vi "Advanced Serial Write and Read.vi"(0 "VISA resource name":refnum<visa-resource-name>="COM1", 1 "baud rate":u32=9600, 3 "bytes to read":u32=1000, 4 "data bits":u16=8 min=5 max=8 step=1, 5 "parity":u16(ring) items=["None", "Odd", "Even", "Mark", "Space"], 7 "stop bits":u16(ring)=10 items=["1.0"=10, "1.5"=15, "2.0"=20], 9 "XON Character":u8=17 format="%.0x", 13 "string to write":string="*IDN?", 14 "XOFF Character":u8=19 format="%.0x", 15 "timeout (ms)":u32=10000, 17 "write":bool=TRUE, 21 "End read on termination character?":bool=TRUE, 24 "termination char\n(0xA = '\\n' = LF)":u8=10 format="%.0x", 25 "Input\nbuffer size":u32=4096, 26 "read":bool=TRUE) -> (20 "read string":string)   [LabVIEW 2011]
doc: "The Advanced Serial Read and Write example performs a Serial Port Read, a Serial Port Write, or a combination of these actions while setting some advanced serial features like buffer size, termination characters, and XON/XOFF flow control. The user selects the actions (read or write) on the front panel. If both are selected, the VI will write the data first, read the data and then close the VISA session that is opened to the port. \n\nThe parameters set for the serial port must match the parameters of the connected instrument or device. In this example, the bytes to read parameter specifies the number of bytes that the serial port reads. If there were more bytes at the port than the number specified in bytes to read, those bytes would not be read. Also, if you specify to read more bytes than the number of bytes actually read, you might receive a timeout error message.\n\nINSTRUCTIONS:\n1) Select the serial resource and configuration parameters (baud rate, data bits, parity, stop bits, flow control).\n2) Termination character can be enabled and set. Also, set the required input buffer size prior to running the example.\n3) Select the operations to be performed. \n4) Connect the serial port to your device. If no device is available, perform a loopback test by doing one of the following. Short pins 2 and 3 on a RS-232 cable or short pin 4 to pin 8 and pin 5 to pin 9 on a RS-485/422 cable. \n5) Run the VI to see the data read. (The \"read string\" will match the \"string to write\" if a loopback test was performed.)\n\nThis example exposes several advanced features that you may need for your application. Not all applications need all the features shown in this example. The input buffer size is likely an important setting that you want to control in your application. This example expands upon the flow control option for XON and XOFF, allowing the user to choose those control characters. The timeout parameter has been brought to the front panel so a user can specify the time period the VISA Read will wait for the number of bytes to read before timing out. Also, the user has several controls for the termination character, which is discussed later.\n\nNote that you can press the write and read buttons and change the bytes to read parameters on the fly, while the example is running. However, you must stop the example to change the other configuration parameters after the example has started running, and then run again.\n\nSet the I/O buffer size slightly higher the amount of data you expect to receive. This is very important for applications that don't use flow control, as you may lose characters if the receive buffer overflows.\n\nSetting the timeout period ensures that the operation returns with a timeout error if the operation cannot be performed in the specified time period. \n\nSome devices require a termination character in order to identify the end of command strings. Some devices send a termination character to signify the end of data to be read. \n\nThis example shows how you can end the Read operation once a termination character is detected in the buffer and/or append a termination character at the end of the Write data. To enable the Read to end on a termination character, use the VISA Configure Serial Port or use the VISA Properties Serial End Mode for Reads, Termination Character Enable, and Termination Character. To end the Write with a termination character, use the VISA Properties Serial End Mode for Writes, the Send End Enable, and Termination Character. In this example, the same termination character is used for both the Read and the Write. You can specify two different characters for your application, if desired.\n\nYour application may require specific characters for the XON/XOFF Flow Control. You can specify these characters with the VISA Properties Flow Control XOFF Character and Flow Control XON Character. Note that if the standard XON and XOFF characters are used, then decimal 17 and 19 are unavailable for data values. Remember that using flow control and setting an adequate buffer size allow you to prevent buffer overflows."
uses:
  <vilib>/Instr/_visa.llb/VISA Configure Serial Port (Instr).vi
panel:
  out "actual bytes read":u32
  in  "stop":bool
  in  "flow control":u16(ring) items=["None"=0, "XON/XOFF"=1, "RTS/CTS"=2, "DTR/DSR"=4]
  in  "End write with termination character?":bool=TRUE
  # "On Windows/Linux, consider using the Instrument Driver Finder (Help>>Find Instrument Drivers) to search for an instrument driver for your instrument."
  # "Select the serial resource and the operations to be performed.  If all are selected, the VI will write the data first, read data and then close the VISA session that is opened to the port.  This VI will wait until the specified number of bytes is received at the port, until the timeout period is met, or until a termination character is received.  The default termination character in this example is the Line Feed ( ASCII 0xA, '\\n' ).  Also, set the required input buffer size prior to running the example.\nNote: The example loops until the STOP button is pressed."
  # "For additional information select File >> VI Properties >> Documentation"
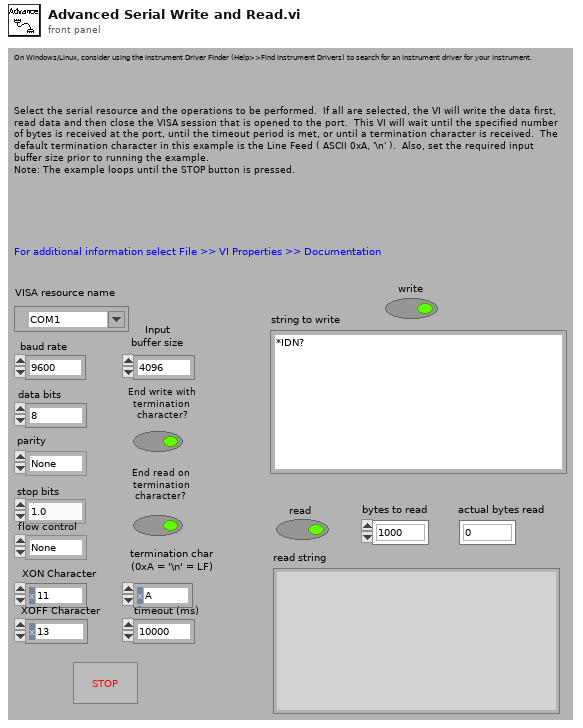
[diagram p1: front panel]
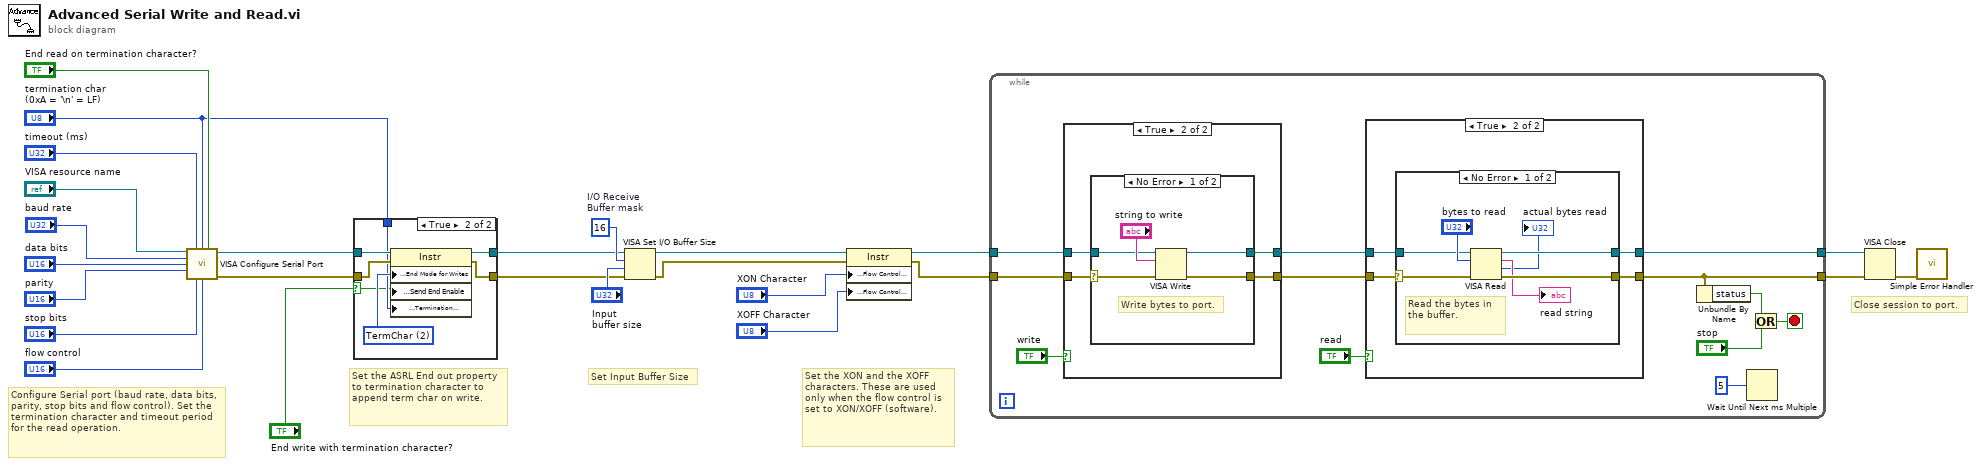
[diagram p0: block diagram]
diagram:
  w18 = u16 16  # I/O Receive Buffer mask
  # "Set the XON and the XOFF characters. These are used only when the flow control is set to XON/XOFF (software)."
  # "Configure Serial port (baud rate, data bits, parity, stop bits and flow control). Set the termination character and timeout period for the read operation."
  # "Set Input Buffer Size"
  # "Set the ASRL End out property to termination character to append term char on write."
  # "Close session to port."
  n1 = call-poly "VISA Configure Serial Port"("VISA resource name"="VISA resource name", "timeout (10sec)"="timeout (ms)", "termination char\n(0xA = '\\n' = LF)"="termination char\n(0xA = '\\n' = LF)", "Enable Termination\nChar (T)"="End read on termination character?", "baud rate (9600)"="baud rate", "data bits (8)"="data bits", "parity (0:none)"="parity", "stop bits (10: 1 bit)"="stop bits", "flow control (0:none)"="flow control") -> ("VISA resource name out"=w4:refnum<visa-resource-name>, "error out"=w7:errorcluster)  [unwired: 1 in, 4 out]
  n2 = case shown="True" "End write with termination character?" {
    selector: "End write with termination character?" -> [_ w28]
    tunnel: w4 -> [w26 w34]
    tunnel: w7 -> [w27 w33]
    tunnel: [w26 w32] -> w5
    tunnel: [w27 w31] -> w6
    tunnel: "termination char\n(0xA = '\\n' = LF)" -> [_ w29]
    frame False {
    }
    frame True {
      w30 = u16 2 items=["None", "LastBit", "TermChar", "Break"] ("Serial Settings:Serial End Mode for Writes")
      n3 = property on="Property Node" class="Instr"(reference=w34, error in=w33, "Serial Settings:End Mode for Writes"=w30, "Message Based Settings:Send End Enable"=w28, "Message Based Settings:Termination Character"=w29) -> (reference out=w32:refnum<visa-resource-name>, error out=w31:errorcluster)
    }
  }
  n4 = VISA Set I/O Buffer Size(VISA resource name=w5, mask (16)=w18, size (4096)="Input\nbuffer size", error in (no error)=w6) -> (VISA resource name out=w13:refnum<visa-resource-name>, error out=w12:errorcluster)
  n5 = property class="Instr"(reference=w13, error in=w12, "Serial Settings:Flow Control XON Character"="XON Character", "Serial Settings:Flow Control XOFF Character"="XOFF Character") -> (reference out=w3:refnum<visa-resource-name>, error out=w9:errorcluster)
  n6 = while {
    tunnel: w9 -> [w39]
    tunnel: w3 -> [w40]
    tunnel: [w38] -> w2
    tunnel: [w37] -> w1
    stop <- w36 stop-if-true
    n7 = case shown="True" "write" {
      tunnel: [w48 w52] -> w43
      tunnel: [w47 w51] -> w42
      tunnel: w40 -> [w48 w50]
      tunnel: w39 -> [w47 w49]
      frame False {
      }
      frame True {
        n8 = case shown="No Error" w49 {
          selector: w49 -> [w53 w59]
          tunnel: [w57 w58] -> w52
          tunnel: [w56 w59] -> w51
          tunnel: w50 -> [w54 w58]
          frame No Error {
            # "Write bytes to port."
            n9 = VISA Write(VISA resource name=w54, write buffer="string to write", error in (no error)=w53) -> (VISA resource name out=w57:refnum<visa-resource-name>, error out=w56:errorcluster)  [unwired: 1 out]
          }
          frame Error {
          }
        }
      }
    }
    n10 = case shown="True" "read" {
      tunnel: w42 -> [w60 w63]
      tunnel: w43 -> [w61 w62]
      tunnel: [w60 w65] -> w37
      tunnel: [w61 w64] -> w38
      frame False {
      }
      frame True {
        n11 = case "Read bytes from port." shown="No Error" w63 {
          selector: w63 -> [w67 w73]
          tunnel: [w71 w73] -> w65
          tunnel: [w72 w74] -> w64
          tunnel: w62 -> [w68 w74]
          frame No Error {
            # "Read the bytes in the buffer."
            n12 = VISA Read(VISA resource name=w68, byte count="bytes to read", error in (no error)=w67) -> (VISA resource name out=w72:refnum<visa-resource-name>, read buffer=→"read string":string, return count=→"actual bytes read":u32, error out=w71:errorcluster)
          }
          frame Error {
            # "Error occurred \nreading Bytes at \nSerial Port"
          }
        }
      }
    }
    n13 = Unbundle By Name(w37) -> ("status"=w44:bool)
    n14 = Wait Until Next ms Multiple(millisecond multiple=u32 5) -> ()  [unwired: 1 out]
    n15 = Or(x=w44, y="stop") -> (x .or. y?=w36:bool)
  }
  n16 = VISA Close(VISA resource name=w2, error in (no error)=w1) -> (error out=w23:errorcluster)
  n17 = call <vilib>:"Simple Error Handler.vi"("error in (no error)"=w23) -> ()  [unwired: 1 in, 8 out]
